vi "Read Safe Temperature Range.vi"(11 "VacuumLines in":refnum<class "VacuumLines.lvclass">) -> (2 "Safe Temperature Range":cluster{"min":dbl, "max":dbl}={"min"=0.0, "max"=40.0}, 3 "VacuumLines out":refnum<class "VacuumLines.lvclass">)   [LabVIEW 2016, in "Hardware.lvlib" / "VacuumLine.lvlib" / "VacuumLines.lvclass"]
uses:
  <userlib>/Common Components/Hardware/Abstract System/VacuumLine/VacuumLines/VacuumLines.lvclass
  <userlib>/Common Components/Hardware/Abstract System/VacuumLine/VacuumLines/VacuumLines.lvclass/VacuumLines.ctl
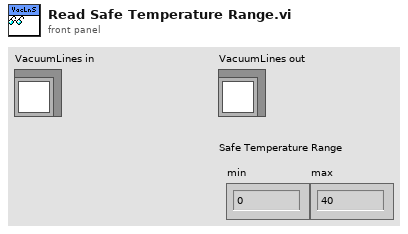
[diagram p1: front panel]
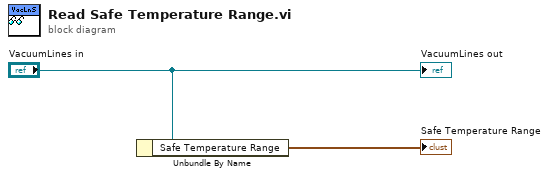
[diagram p0: block diagram]
diagram:
  n1 = Unbundle By Name("VacuumLines in") -> ("Safe Temperature Range"=→"Safe Temperature Range":cluster{"min":dbl, "max":dbl})
  "VacuumLines out" <- "VacuumLines in"
